vi "Init.vi"(8 "error in (no error)":errorcluster, 9 "Ti Cathode":i8=-1, 10 "Name":string, 11 "Sample in":bool) -> (0 "error out":errorcluster, 3 "Sample out":refnum<class "Sample.lvclass">)   [LabVIEW 2015, in "Sample.lvclass"]
uses:
  Sample.lvclass
  Sample.lvclass/Sample.ctl
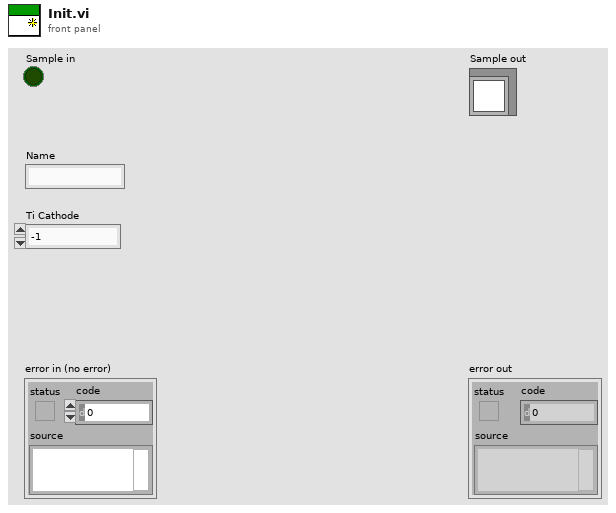
[diagram p1: front panel]
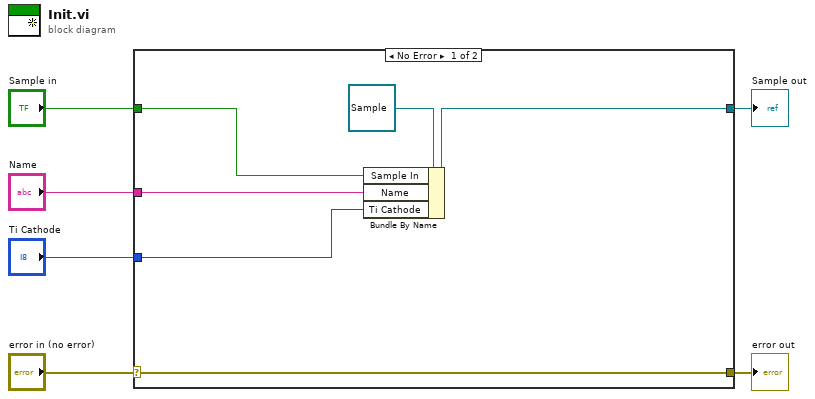
[diagram p0: block diagram]
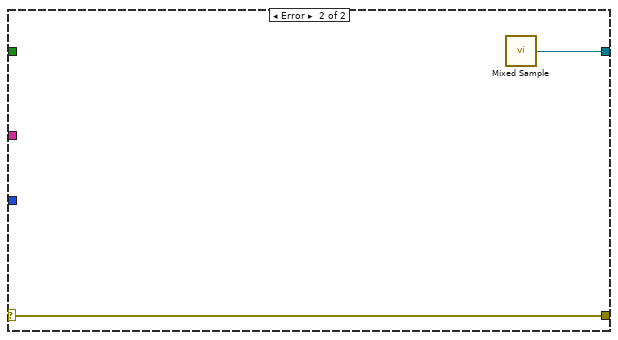
[diagram p2: hidden frame]
diagram:
  n1 = case shown="No Error" "error in (no error)" {
    selector: "error in (no error)" -> [w12 w14]
    tunnel: [w12 w14] -> w5
    tunnel: [w11 w13] -> w1
    tunnel: "Sample in" -> [w7 _]
    tunnel: "Name" -> [w10 _]
    tunnel: "Ti Cathode" -> [w9 _]
    frame No Error {
      n2 = Bundle By Name(cluster=refnum<class "Sample.lvclass"> refnum ("Sample out"), "Sample In"=w7, "Name"=w10, "Ti Cathode"=w9) -> (w11:refnum<class "Sample.lvclass">)
    }
    frame Error {
      n3 = call "Mixed Sample.vi"() -> ("Mixed Sample (Sample In: true)"=w13:refnum<class "Sample.lvclass">)
    }
  }
  "error out" <- w5
  "Sample out" <- w1
